vi "2 midpoint.vi"(9 "UTM 2":T1, 11 "UTM 1":T1) -> (2 "Midpoint":T1)   [LabVIEW 2011]
uses:
  2 Typedefs/UTM Location.ctl
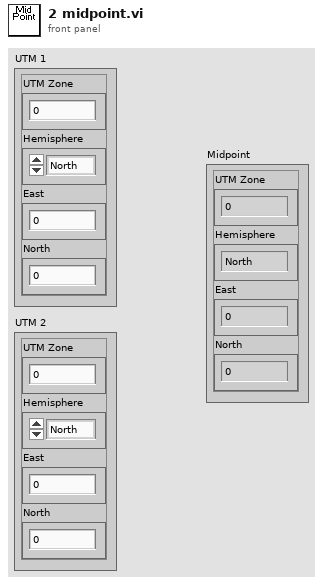
[diagram p1: front panel]
types:
  T1 = typedef "UTM Location.ctl" = cluster{"UTM Zone":dbl, "Hemisphere":enum16{"North", "South"}, "East":dbl, "North":dbl}
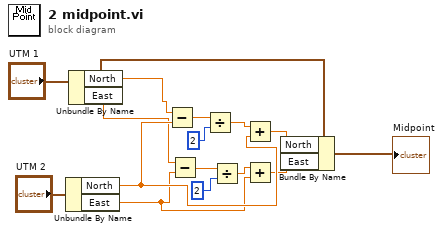
[diagram p0: block diagram]
diagram:
  n1 = Unbundle By Name("UTM 2") -> ("North"=w9:dbl, "East"=w8:dbl)
  n2 = Unbundle By Name("UTM 1") -> ("North"=w5:dbl, "East"=w4:dbl)
  n3 = Subtract(x=w5, y=w9) -> (x-y=w14:dbl)
  n4 = Subtract(x=w4, y=w8) -> (x-y=w15:dbl)
  n5 = Divide(x=w14, y=2) -> (x/y=w10:dbl)
  n6 = Divide(x=w15, y=2) -> (x/y=w11:dbl)
  n7 = Add(x=w10, y=w9) -> (x+y=w6:dbl)
  n8 = Add(x=w11, y=w8) -> (x+y=w7:dbl)
  n9 = Bundle By Name(cluster="UTM 1", "North"=w6, "East"=w7) -> (→"Midpoint":T1)
